vi "Compute Colour Pair.vi"(5 "Fractional Scale Upper":sgl=0.1, 7 "Fractional Scale Lower":sgl=0.1, 8 "error in (no error)":errorcluster, 11 "Starting Colour":u32(colorbox)) -> (0 "error out":errorcluster, 3 "Colour Pair":T1)   [LabVIEW 2020, in "image.lvlib"]
doc: "Compute a colour which is fractionally lighter and darker than the starting colour."
uses:
  image.lvlib
  In-Range Image Colour Range.ctl
  common/common.lvlib
  common/bin/gartoolkit_32-1.dll
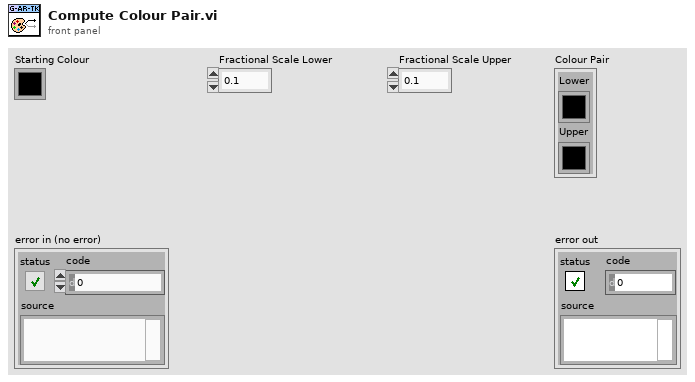
[diagram p1: front panel]
types:
  T1 = typedef "image.lvlib/In-Range Image Colour Range.ctl" = cluster{"Lower":u32, "Upper":u32}
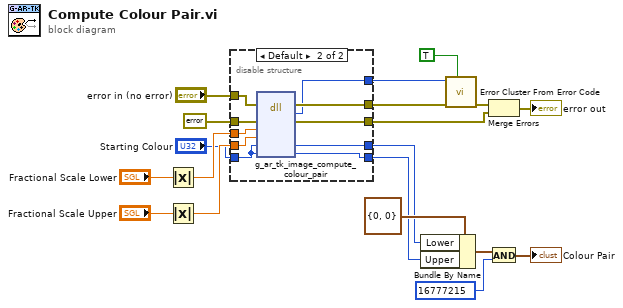
[diagram p0: block diagram]
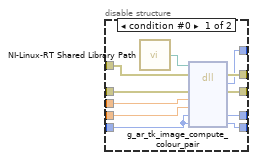
[diagram p2: hidden frame]
diagram:
  n1 = Absolute Value(x="Fractional Scale Lower") -> (abs(x)=w11:sgl)
  n2 = Absolute Value(x="Fractional Scale Upper") -> (abs(x)=w10:sgl)
  n3 = disable-structure shown="Default" {
    disable-tunnel: "error in (no error)" -> [w30 w40]
    disable-tunnel: errorcluster {"status"=FALSE, "code"=0, "source"=""} ("error constant") -> [w29 w39]
    disable-tunnel: w11 -> [w28 w38]
    disable-tunnel: w10 -> [w27 w37]
    disable-tunnel: "Starting Colour" -> [w26 w36]
    disable-tunnel: [w25 w35] -> w8
    disable-tunnel: [w24 w34] -> w7
    disable-tunnel: [w23 w33] -> w6
    disable-tunnel: [w22 w32] -> w5
    disable-tunnel: [w21 w31] -> w4
    frame condition #0 {
      n4 = call "NI-Linux-RT Shared Library Path.vi"() -> ("Path"=w20:path)
      n5 = dll-call lib="?" fn="g_ar_tk_image_compute_colour_pair" ("g_ar_toolkit.*.*:g_ar_tk_image_get_text_size")(path in=w20, error in=w30, "error"=w29, "Fractional_Scale_Lower"=w28, "Fractional_Scale_Upper"=w27, "Darker"=w26, "Lighter"=w26) -> (error out=w25:errorcluster, w24:i32, "error"=w23:errorcluster, "Darker"=w22:u32, "Lighter"=w21:u32)  [unwired: 3 in, 1 out]
    }
    frame condition #1 (active) {
      n6 = dll-call lib="C:/serenial/lib/g-augmented-reality-toolkit/LabVIEW/common/bin/gartoolkit_*-1.*" fn="g_ar_tk_image_compute_colour_pair" ("g_ar_toolkit.*.*:g_ar_tk_image_get_text_size")(error in=w40, "error"=w39, "Fractional_Scale_Lower"=w38, "Fractional_Scale_Upper"=w37, "Darker"=w36, "Lighter"=w36) -> (error out=w35:errorcluster, w34:i32, "error"=w33:errorcluster, "Darker"=w32:u32, "Lighter"=w31:u32)  [unwired: 4 in, 1 out]
    }
  }
  n7 = Bundle By Name(cluster=T1 {"Lower"=0, "Upper"=0} ("In-Range Image Colour Range"), "Lower"=w5, "Upper"=w4) -> (w15:T1)
  n8 = call <vilib>:"Error Cluster From Error Code.vi"("show call chain? (False)"=TRUE, "error in (no error)"=w8, "error code (0)"=w7) -> ("error out"=w18:errorcluster)  [unwired: 6 in]
  n9 = Merge Errors(w18, w6) -> (→"error out":errorcluster)
  n10 = And(x=w15, y=u32 16777215) -> (x .and. y?=→"Colour Pair":T1)
